vi "SendDashCAN.vi"(8 "CAN E":errorcluster, 9 "y":i32=2, 10 "Enable Dash CAN":bool, 11 "CAN In":refnum<k20>) -> (0 "error out":errorcluster, 2 "Enable Dash CAN Next Run":bool=TRUE, 3 "interface object out":refnum<k20>)   [LabVIEW 2014]
uses:
  Global Data.vi
  NDashPage.ctl
  <vilib>/RioEmbeddedCAN/RioEmbeddedCAN.llb/CANFrameControl.ctl
  <vilib>/RioEmbeddedCAN/RioEmbeddedCAN.llb/CANWaitTransmitComplete.vi
  Sgl_to_Half_Prec_Array.vi
  <resource>/objmgr/RioEmbeddedCANInterface.rc
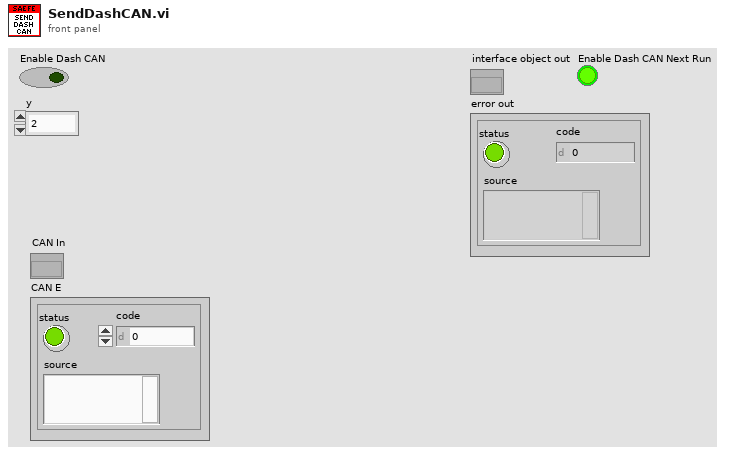
[diagram p1: front panel]
types:
  T1 = typedef "CANFrameControl.ctl" = cluster{"identifier":u32, "extended?":bool, "type":u8, "payload":u8[]}
  T2 = typedef "NDashPage.ctl" = enum16{"Primary", "Warning", "WaitingForCAN", "InPits"}
  T3 = typedef "FPGA Telemetry.ctl" = cluster{"sbRIO":cluster{"Supply Voltage (V)":fxp<+/-,25,6>, "FPGA LED":bool, "Chassis Temperature":fxp<+/-,16,9>}, "Throttles":cluster{"Throttles Consistent?":bool, "Throttles In Range?":bool, "Average Throttle (%)":fxp<+/-,29,18>, "Throttle 2 (V)":fxp<+/-,24,5>, "Throttle 2 (%)":fxp<+/-,27,18>, "Throttle 1 (V)":fxp<+/-,24,5>, "Throttle 1 (%)":fxp<+/-,27,18>, "Throttle 2 Max":fxp<+,16,4>, "Throttle 2 Min":fxp<+,16,4>, "Throttle 1 Max":fxp<+,16,4>, "Throttle 1 Min":fxp<+,16,4>, "Unscaled Throttle 2 Percent":fxp<+/-,16,1>, "Unscaled Throttle 1 Percent":fxp<+/-,16,1>}, "Loads & Shutdown":T4, "Motor Controller":cluster{"Motor Controller Dash Switch":bool, "Motor Controller Enable":bool}, "Sensors":cluster{"RL Tick Period":u32, "RR Tick Period":u32, "FR Tick Period":u32, "FL Tick Period":u32, "RR Shock (V)":fxp<+/-,24,5>, "RL Shock (V)":fxp<+/-,24,5>, "FR Shock (V)":fxp<+/-,24,5>, "FL Shock (V)":fxp<+/-,24,5>, "RR Stopped":bool, "RL Stopped":bool, "FR Stopped":bool, "FL Stopped":bool, "Steering Wheel Middle":fxp<+/-,26,5>, "Steering Wheel Angle (degrees)":fxp<+/-,31,13>, "High Current OK?":bool, "Low Current OK?":bool, "Rear BPS OK?":bool, "Front BPS OK?":bool, "Rear BP (psi)":fxp<+/-,27,16>, "Front BP (psi)":fxp<+/-,27,16>, "High Current (A)":fxp<+/-,24,15>, "Low Current (A)":fxp<+/-,24,15>, "RR State":bool, "RL State":bool, "FR State":bool, "FL State":bool, "5V Supply":fxp<+/-,24,5>}, "CPU Load":cluster{"Total (%)":dbl, "Time Critical (%)":dbl, "Timed Structures (%)":dbl, "High (%)":dbl, "Above Normal (%)":dbl, "Normal (%)":dbl, "Background (%)":dbl, "Idle (%)":dbl, "ISR (%)":dbl}, "Vehicle Status":cluster{"BMS Status":T6, "MC Status":T6, "Shutdown Status":T6, "sbRIO Status":T6, "Vehicle Status":T6, "Shutdown State":T9, "AIR Status":T10, "Remote Return to Pits":bool, "Reason for Shutdown":T11, "MC State Machine Status":T12}, "iPhone HF Data":cluster{"Accel X":dbl, "Accel Y":dbl, "Accel Z":dbl, "Gyro X":dbl, "Gyro Y":dbl, "Gyro Z":dbl}, "iPhone LF Data":cluster{"Lat":dbl, "Long":dbl, "Speed":dbl}}
  T4 = typedef "FPGA Loads and Shutdown.ctl" = cluster{"RTDS Enable":bool, "TSMS In Status":bool, "Positive AIR Enable":bool, "cRIO Shutdown 2":bool, "cRIO Shutdown 1":bool, "TSMS Out Status":bool, "Coolant Pump":bool, "BMS OK":bool, "IMD In":bool, "BSPD In":bool, "Brake Light Out":bool, "Green LED":T5, "Yellow LED":T5, "Red LED":T5}
  T5 = typedef "Dash LED Status.ctl" = enum16{"Off", "Flashing", "On"}
  T6 = typedef "Subsystem Status.ctl" = cluster{"eStatusSeverity":T7, "NValue":sgl, "CMessage":T8, "bNotOK":bool}
  T7 = typedef "Subsystem Status Severity.ctl" = enum16{"Okay", "Short Warning", "Long Warning", "Return to Pits", "Error", "Danger"}
  T8 = typedef "Subsystem Status Message.ctl" = enum16{"ControllerTemperature", "MotorTemperature", "BatteryTemperature", "BatteryLowVoltage", "LVBattery", "sbRIOTemperature", "Precharge", "BSPD", "IMD", "RemoteReturnToPits", "EStopInterrupted", "NoCellComms", "MCOverSpeed", "MCOverCurrent", "MCOverVoltage", "MCInverterOverTemp", "MCDirectionCommand", "MCInverterTimeout", "MCDesatFault", "MCHWOverCurrent", "MCUnderVoltage", "MCCommandMessageLost", "MotorOverTemp", "MCModAOverTemp", "MCModBOverTemp", "MCModCOverTemp", "MCPCBOverTemp", "MCGateDrv1OverTemp", "MCDateDrv2OverTemp", "MCCurrentSensorFault", "MCResolverNotConnected", "ShutdownLatchTripped", "UnknownBMS", "RemoteEmergency"}
  T9 = typedef "Shutdown State Machine.lvsc/State.ctl" = enum16{"NI.SC.Initial", "NI.SC.History", "NI.SC.ShallowHistory", "NI.SC.Terminal", "Coolant Pump Started/AIR's On", "AIRs On", "Precharge", "TSMS Off"}
  T10 = typedef "AIR Status.ctl" = enum16{"Off", "Precharge", "On"}
  T11 = typedef "Reason for Shutdown.ctl" = enum16{"None", "BMS", "Shutdown", "sbRIO", "MC", "Remote"}
  T12 = typedef "MC State Machine.lvsc/State.ctl" = enum16{"NI.SC.Initial", "NI.SC.History", "NI.SC.ShallowHistory", "NI.SC.Terminal", "Let Current Drop then Disable AIR's", "Enabled", "Disabled"}
  T13 = typedef "BMS Telemetry.ctl" = cluster{"Ignition":bool, "Charger Mains":bool, "Fast Charge":bool, "Simple Charger Enabled":bool, "Car State":enum16{"Off", "On, Not Charging", "Charging", "Charging Finished", "Charging Error"}, "Charging State":enum16{"Disconnected", "Pre-charging", "Main Charging", "Balancing", "Charging Finished OK", "Charging Error"}, "Charging Stage Duration":u16, "Last Charging Error":enum16{"No Error", "Cell Voltage Too Low", "No Comm from Cells so can't start", "Maximum charging stage duration expired", "No Comm from Cels so can't balande", "Cannot set balancing voltage", "Cell temps too high", "No Comms so can't determine temp", "# of Cells Mismatch", "Cells Overvoltage", "Cell Protection Event occured."}, "Number of Detected Cells":u8, "Under-Voltage":bool, "Over-Voltage":bool, "Overheat":bool, "Leakage":bool, "No Cell Comms":bool, "Low Voltage":bool, "High Temperature":bool, "Min Cell V":dbl, "Max Cell V":dbl, "Mean Cell V":dbl, "Total V":dbl, "Min Cell t":dbl, "Max Cell t":dbl, "Mean Cell t":dbl, "Cell Voltages":cluster{"[0]":dbl, "[1]":dbl, "[2]":dbl, "[3]":dbl, "[4]":dbl, "[5]":dbl, "[6]":dbl, "[7]":dbl, "[8]":dbl, "[9]":dbl, "[10]":dbl, "[11]":dbl, "[12]":dbl, "[13]":dbl, "[14]":dbl, "[15]":dbl, "[16]":dbl, "[17]":dbl, "[18]":dbl, "[19]":dbl, "[20]":dbl, "[21]":dbl, "[22]":dbl, "[23]":dbl, "[24]":dbl, "[25]":dbl, "[26]":dbl, "[27]":dbl, "[28]":dbl, "[29]":dbl, "[30]":dbl, "[31]":dbl, "[32]":dbl, "[33]":dbl, "[34]":dbl, "[35]":dbl, "[36]":dbl, "[37]":dbl, "[38]":dbl, "[39]":dbl, "[40]":dbl, "[41]":dbl, "[42]":dbl, "[43]":dbl, "[44]":dbl, "[45]":dbl, "[46]":dbl, "[47]":dbl, "[48]":dbl, "[49]":dbl, "[50]":dbl, "[51]":dbl, "[52]":dbl, "[53]":dbl, "[54]":dbl, "[55]":dbl, "[56]":dbl, "[57]":dbl, "[58]":dbl, "[59]":dbl, "[60]":dbl, "[61]":dbl, "[62]":dbl, "[63]":dbl, "[64]":dbl, "[65]":dbl, "[66]":dbl, "[67]":dbl, "[68]":dbl, "[69]":dbl, "[70]":dbl}, "Cell Temps":cluster{"[0]":dbl, "[1]":dbl, "[2]":dbl, "[3]":dbl, "[4]":dbl, "[5]":dbl, "[6]":dbl, "[7]":dbl, "[8]":dbl, "[9]":dbl, "[10]":dbl, "[11]":dbl, "[12]":dbl, "[13]":dbl, "[14]":dbl, "[15]":dbl, "[16]":dbl, "[17]":dbl, "[18]":dbl, "[19]":dbl, "[20]":dbl, "[21]":dbl, "[22]":dbl, "[23]":dbl, "[24]":dbl, "[25]":dbl, "[26]":dbl, "[27]":dbl, "[28]":dbl, "[29]":dbl, "[30]":dbl, "[31]":dbl, "[32]":dbl, "[33]":dbl, "[34]":dbl, "[35]":dbl, "[36]":dbl, "[37]":dbl, "[38]":dbl, "[39]":dbl, "[40]":dbl, "[41]":dbl, "[42]":dbl, "[43]":dbl, "[44]":dbl, "[45]":dbl, "[46]":dbl, "[47]":dbl, "[48]":dbl, "[49]":dbl, "[50]":dbl, "[51]":dbl, "[52]":dbl, "[53]":dbl, "[54]":dbl, "[55]":dbl, "[56]":dbl, "[57]":dbl, "[58]":dbl, "[59]":dbl, "[60]":dbl, "[61]":dbl, "[62]":dbl, "[63]":dbl, "[64]":dbl, "[65]":dbl, "[66]":dbl, "[67]":dbl, "[68]":dbl, "[69]":dbl, "[70]":dbl}}
  T14 = typedef "MC Temp 3.ctl" = cluster{"RTD #4":dbl, "RTD #5":dbl, "Motor (C)":dbl, "T-Shudder":dbl}
  T15 = typedef "MC Temp 1.ctl" = cluster{"IGBT A (C)":dbl, "IGBT B (C)":dbl, "IGBT C (C)":dbl, "Gate Driver (C)":dbl}
  T16 = typedef "MC Temp 2.ctl" = cluster{"Control Board (C)":dbl, "RTD #1":dbl, "RTD #2":dbl, "RTD #3":dbl}
  T17 = typedef "MC Current.ctl" = cluster{"I-Phase A":dbl, "I-Phase B":dbl, "I-Phase C":dbl, "I-Battery":dbl}
  T18 = typedef "MC Voltage.ctl" = cluster{"V-Phase AB":dbl, "V-Phase BC":dbl, "V-Output":dbl, "V-Battery":dbl}
  T19 = typedef "MC Position.ctl" = cluster{"Motor Angle":dbl, "Motor Speed":dbl, "Electrical Output Freq.":dbl, "Delta Resolver Filt.":dbl}
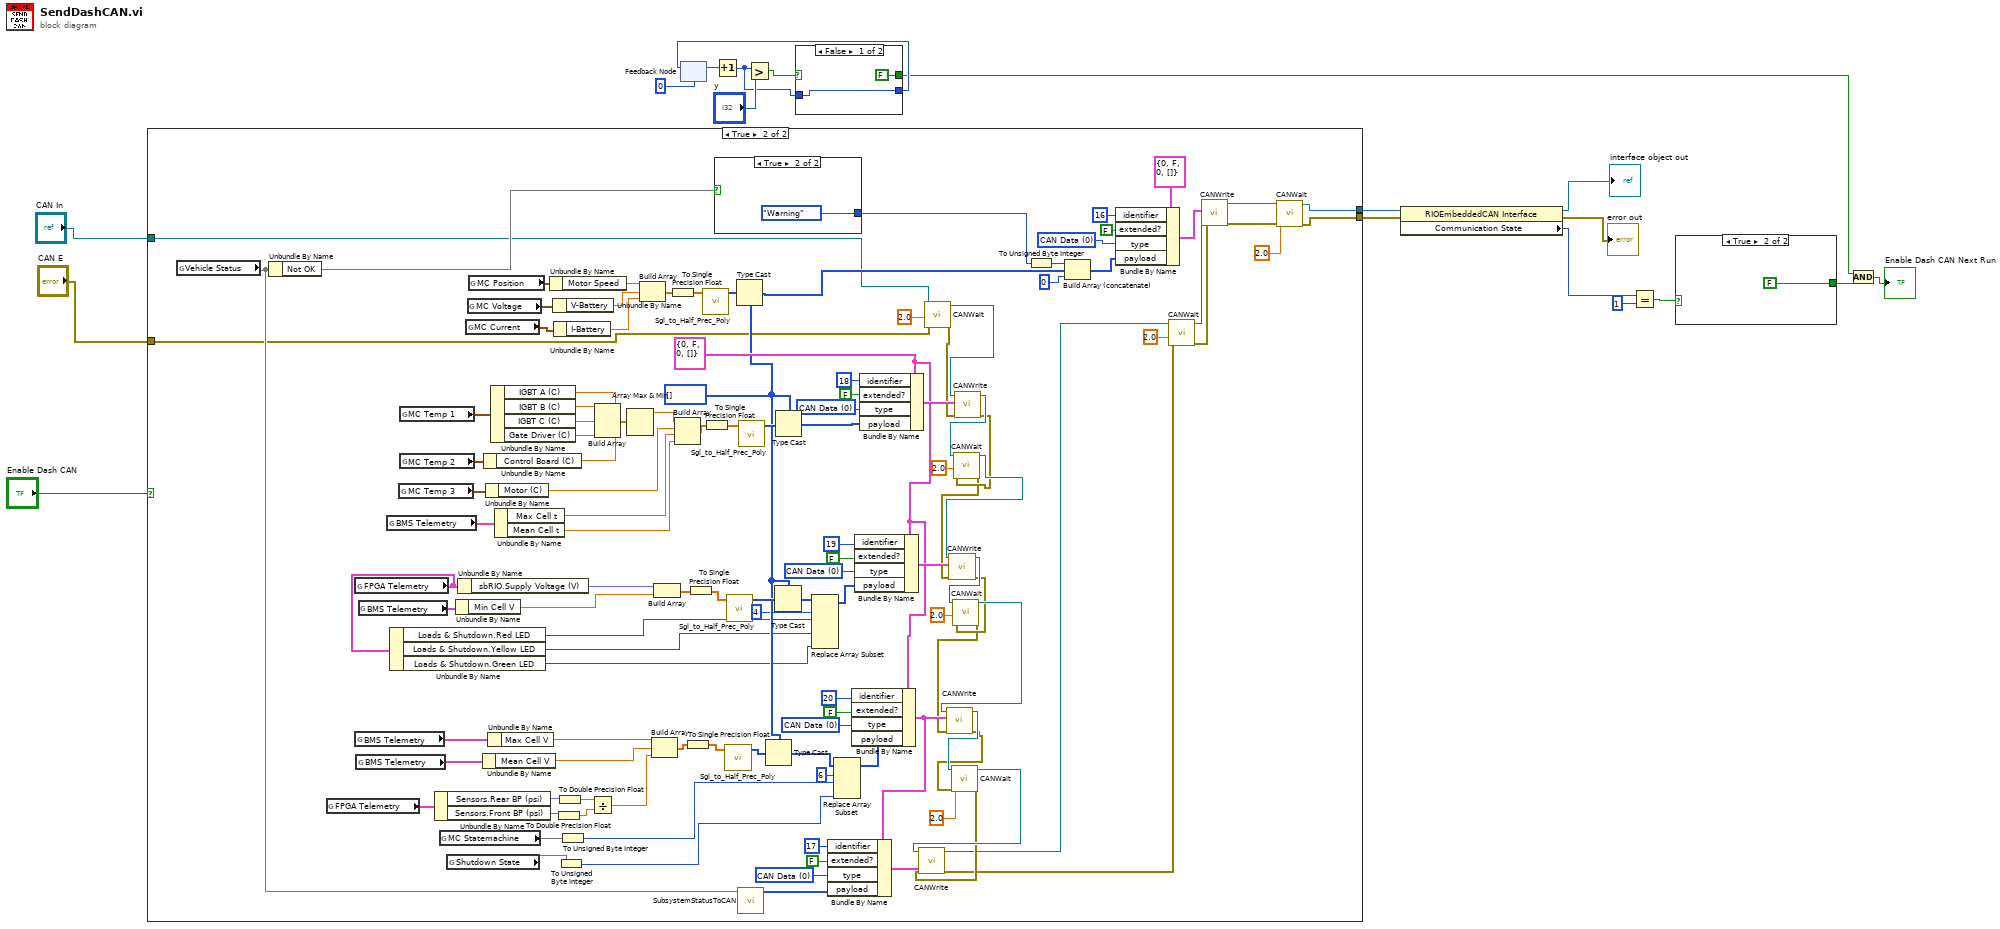
[diagram p0: block diagram]
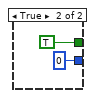
[diagram p2: hidden frame]
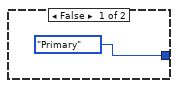
[diagram p4: hidden frame]
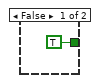
[diagram p5: hidden frame]
diagram:
  n1 = case shown="True" "Enable Dash CAN" {
    tunnel: [w21 w32] -> w16
    tunnel: [w20 w31] -> w15
    tunnel: "CAN In" -> [w21 w30]
    tunnel: "CAN E" -> [w20 w29]
    frame False {
    }
    frame True {
      w105 = u8 0 items=["CAN Data", "CAN Remote"] ("type")
      w115 = u8 0 items=["CAN Data", "CAN Remote"] ("type")
      w118 = u8 0 items=["CAN Data", "CAN Remote"] ("type")
      w97 = T1 {"identifier"=0, "extended?"=FALSE, "type"=0, "payload"=[]} ("CAN frame")
      w68 = u8[] []
      w132 = u8 0 items=["CAN Data", "CAN Remote"] ("type")
      w140 = u8 0 items=["CAN Data", "CAN Remote"] ("type")
      n2 = global read "Global Data.vi" "Vehicle Status"() -> (w82)
      n3 = Unbundle By Name(w82) -> ("Not OK"=w81)
      n4 = global read "Global Data.vi" "FPGA Telemetry"() -> (w64:T3)
      n5 = global read "Global Data.vi" "FPGA Telemetry"() -> (w28:T3)
      n6 = global read "Global Data.vi" "BMS Telemetry"() -> (w102:T13)
      n7 = global read "Global Data.vi" "BMS Telemetry"() -> (w100:T13)
      n8 = global read "Global Data.vi" "BMS Telemetry"() -> (w110:T13)
      n9 = global read "Global Data.vi" "BMS Telemetry"() -> (w80:T13)
      n10 = Unbundle By Name(w28) -> ("Loads & Shutdown.Red LED"=w24:T5, "Loads & Shutdown.Yellow LED"=w23:T5, "Loads & Shutdown.Green LED"=w22:T5)
      n11 = global read "Global Data.vi" "MC Temp 3"() -> (w120:T14)
      n12 = global read "Global Data.vi" "MC Temp 1"() -> (w129:T15)
      n13 = global read "Global Data.vi" "MC Temp 2"() -> (w128:T16)
      n14 = Unbundle By Name(w64) -> ("Sensors.Rear BP (psi)"=w63:fxp<+/-,27,16>, "Sensors.Front BP (psi)"=w62:fxp<+/-,27,16>)
      n15 = global read "Global Data.vi" "MC Statemachine"() -> (w59)
      n16 = global read "Global Data.vi" "Shutdown State"() -> (w58)
      n17 = Unbundle By Name(w110) -> ("Min Cell V"=w109:dbl)
      n18 = Unbundle By Name(w28) -> ("sbRIO.Supply Voltage (V)"=w111:fxp<+/-,25,6>)
      n19 = global read "Global Data.vi" "MC Current"() -> (w73:T17)
      n20 = global read "Global Data.vi" "MC Voltage"() -> (w75:T18)
      n21 = global read "Global Data.vi" "MC Position"() -> (w77:T19)
      n22 = Unbundle By Name(w100) -> ("Mean Cell V"=w99:dbl)
      n23 = Unbundle By Name(w128) -> ("Control Board (C)"=w123:dbl)
      n24 = Unbundle By Name(w120) -> ("Motor (C)"=w119:dbl)
      n25 = Unbundle By Name(w102) -> ("Max Cell V"=w101:dbl)
      n26 = Unbundle By Name(w129) -> ("IGBT A (C)"=w127:dbl, "IGBT B (C)"=w126:dbl, "IGBT C (C)"=w125:dbl, "Gate Driver (C)"=w124:dbl)
      n27 = Unbundle By Name(w80) -> ("Max Cell t"=w79:dbl, "Mean Cell t"=w78:dbl)
      n28 = Unbundle By Name(w77) -> ("Motor Speed"=w76:dbl)
      n29 = Unbundle By Name(w75) -> ("V-Battery"=w74:dbl)
      n30 = Unbundle By Name(w73) -> ("I-Battery"=w72:dbl)
      n31 = To Double Precision Float(number=w62) -> (double precision float=w61:dbl)
      n32 = To Double Precision Float(number=w63) -> (double precision float=w60:dbl)
      n33 = To Unsigned Byte Integer(number=w58) -> (unsigned 8bit integer=w53:u8)
      n34 = To Unsigned Byte Integer(number=w59) -> (unsigned 8bit integer=w54:u8)
      n35 = Divide(x=w60, y=w61) -> (x/y=w57:dbl)
      n36 = Build Array(w127, w126, w125, w124, w123) -> (w122:dbl[])
      n37 = Array Max & Min(array=w122) -> (max value=w121:dbl)  [unwired: 3 out]
      n38 = Build Array(w76, w74, w72) -> (w71:dbl[])
      n39 = Build Array(w101, w99, w57) -> (w98:dbl[])
      n40 = Build Array(w111, w109) -> (w108:dbl[])
      n41 = To Single Precision Float(number=w71) -> (single precision float=w70:sgl[])
      n42 = Build Array(w121, w119, w79, w78) -> (w112:dbl[])
      n43 = To Single Precision Float(number=w98) -> (single precision float=w86:sgl[])
      n44 = To Single Precision Float(number=w108) -> (single precision float=w88:sgl[])
      n45 = call-poly "Sgl_to_Half_Prec_Poly.vi"("SGL"=w70) -> ("Half"=w69:u16[])  [unwired: 4 in]
      n46 = To Single Precision Float(number=w112) -> (single precision float=w90:sgl[])
      n47 = case shown="True" w81 {
        tunnel: [NDashPage."Primary" ("NDashPage") NDashPage."Warning" ("NDashPage")] -> w137
        frame False {
        }
        frame True {
        }
      }
      n48 = call-poly "Sgl_to_Half_Prec_Poly.vi"("SGL"=w86) -> ("Half"=w85:u16[])  [unwired: 4 in]
      n49 = call-poly "Sgl_to_Half_Prec_Poly.vi"("SGL"=w88) -> ("Half"=w87:u16[])  [unwired: 4 in]
      n50 = Type Cast(type=w68, x=w69) -> (*(type *) &x=w51:u8[])
      n51 = call "SubsystemStatusToCAN.vi"("Subystem Status"=w82) -> ("Array"=w131:u8[])  [unwired: 10 in]
      n52 = call-poly "Sgl_to_Half_Prec_Poly.vi"("SGL"=w90) -> ("Half"=w89:u16[])  [unwired: 4 in]
      n53 = Type Cast(type=w68, x=w85) -> (*(type *) &x=w50:u8[])
      n54 = Type Cast(type=w68, x=w87) -> (*(type *) &x=w27:u8[])
      n55 = Type Cast(type=w68, x=w89) -> (*(type *) &x=w52:u8[])
      n56 = Replace Array Subset(array=w27, new element #1=w24, index #1=4 ("index"), new element #2=w23, new element #3=w22) -> (w26:u8[])  [unwired: 2 in]
      n57 = Replace Array Subset(array=w50, new element #1=w54, index #1=6 ("index"), new element #2=w53) -> (w56:u8[])  [unwired: 1 in]
      n58 = Bundle By Name(cluster=w97, "identifier"=u32 20, "extended?"=FALSE, "type"=w105, "payload"=w56) -> (w47:T1)
      n59 = Bundle By Name(cluster=w47, "identifier"=u32 17, "extended?"=FALSE, "type"=w132, "payload"=w131) -> (w130:T1)
      n60 = Bundle By Name(cluster=w97, "identifier"=u32 19, "extended?"=FALSE, "type"=w115, "payload"=w26) -> (w106:T1)
      n61 = Bundle By Name(cluster=w97, "identifier"=u32 18, "extended?"=FALSE, "type"=w118, "payload"=w52) -> (w107:T1)
      n62 = call-poly <vilib>:"CANWait.vi"("error in (no error)"=w29, "timeout (0 s)"=2.0, "interface object in"=w30) -> ("error out"=w46:errorcluster, "interface object out"=w49:refnum<k20>)  [unwired: 7 in]
      n63 = call <vilib>:"CANWrite.vi"("error in (no error)"=w46, "CAN frame"=w107, "interface object in"=w49) -> ("error out"=w45:errorcluster, "interface object out"=w96:refnum<k20>)  [unwired: 7 in]
      n64 = call-poly <vilib>:"CANWait.vi"("error in (no error)"=w45, "timeout (0 s)"=2.0, "interface object in"=w96) -> ("error out"=w44:errorcluster, "interface object out"=w95:refnum<k20>)  [unwired: 7 in]
      n65 = call <vilib>:"CANWrite.vi"("error in (no error)"=w44, "CAN frame"=w106, "interface object in"=w95) -> ("error out"=w43:errorcluster, "interface object out"=w94:refnum<k20>)  [unwired: 7 in]
      n66 = call-poly <vilib>:"CANWait.vi"("error in (no error)"=w43, "timeout (0 s)"=2.0, "interface object in"=w94) -> ("error out"=w42:errorcluster, "interface object out"=w93:refnum<k20>)  [unwired: 7 in]
      n67 = call <vilib>:"CANWrite.vi"("error in (no error)"=w42, "CAN frame"=w47, "interface object in"=w93) -> ("error out"=w41:errorcluster, "interface object out"=w84:refnum<k20>)  [unwired: 7 in]
      n68 = call-poly <vilib>:"CANWait.vi"("error in (no error)"=w41, "timeout (0 s)"=2.0, "interface object in"=w84) -> ("error out"=w38:errorcluster, "interface object out"=w39:refnum<k20>)  [unwired: 7 in]
      n69 = call <vilib>:"CANWrite.vi"("error in (no error)"=w38, "CAN frame"=w130, "interface object in"=w39) -> ("error out"=w36:errorcluster, "interface object out"=w37:refnum<k20>)  [unwired: 7 in]
      n70 = To Unsigned Byte Integer(number=w137) -> (unsigned 8bit integer=w67:u8)
      n71 = Build Array (concatenate)(w67, w51, u8 0 ("element")) -> (w66:u8[])
      n72 = Bundle By Name(cluster=T1 {"identifier"=0, "extended?"=FALSE, "type"=0, "payload"=[]} ("CAN frame"), "identifier"=u32 16, "extended?"=FALSE, "type"=w140, "payload"=w66) -> (w141:T1)
      n73 = call-poly <vilib>:"CANWait.vi"("error in (no error)"=w36, "timeout (0 s)"=2.0, "interface object in"=w37) -> ("error out"=w40:errorcluster, "interface object out"=w136:refnum<k20>)  [unwired: 7 in]
      n74 = call <vilib>:"CANWrite.vi"("error in (no error)"=w40, "CAN frame"=w141, "interface object in"=w136) -> ("error out"=w34:errorcluster, "interface object out"=w35:refnum<k20>)  [unwired: 7 in]
      n75 = call-poly <vilib>:"CANWait.vi"("error in (no error)"=w34, "timeout (0 s)"=2.0, "interface object in"=w35) -> ("error out"=w31:errorcluster, "interface object out"=w32:refnum<k20>)  [unwired: 7 in]
    }
  }
  n76 = feedback #1(0) -> (w8:i32)
  n77 = Increment(x=w8) -> (x+1=w5:i32)
  n78 = Greater?(x=w5, y="y") -> (0:w6:bool)
  n79 = case shown="False" w6 {
    tunnel: w5 -> [w146 _]
    tunnel: [w146 0] -> w4
    tunnel: [FALSE TRUE] -> w1
    frame False {
    }
    frame True {
    }
  }
  n80 = feedback-in #1(w4) -> ()
  n81 = property class="RIOEmbeddedCAN Interface"(reference=w16, error in=w15) -> (reference out=→"interface object out":refnum<k20>, error out=→"error out":errorcluster, "Communication State"=w19:u32)
  n82 = Equal?(x=w19, y=u32 1) -> (x = y?=w17:bool)
  n83 = case shown="True" w17 {
    tunnel: [TRUE FALSE] -> w3
    frame False {
    }
    frame True {
    }
  }
  n84 = And(x=w1, y=w3) -> (x .and. y?=→"Enable Dash CAN Next Run":bool)
